vi "Acquire Waveform.vi"() -> ()   [LabVIEW 2020]
uses:
  Clients/NW and PSD_client/NW and PSD_client Class/NW and PSD_client.lvclass
panel:
  in  "Start Acquisition":bool
  in  "sine amplitude":dbl=1.0 format="%#.6g"
  in  "sine frequency":dbl=1.0 format="%#.6g"
  in  "sampling info":cluster{"Fs":dbl, "#s":dbl}={"Fs"=1000.0, "#s"=10000.0} {"#s" format="%#.6g"; "Fs" format="%#.6g"}
  out "Waveform":sgl[](graph)
  # "Waveform Parameters"
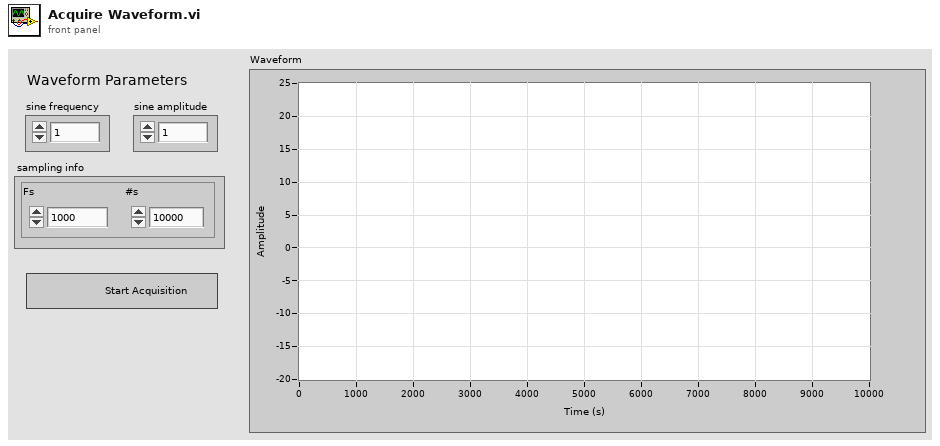
[diagram p1: front panel]
types:
  T1 = cluster{"sine frequency":dbl, "sine amplitude":dbl, "sampling info":cluster{"Fs":dbl, "#s":dbl}, "Start Acquisition?":bool}
  T2 = typedef "NW and PSD_client.lvlib/NW and PSD_client.lvclass/example_SignalData_Data.ctl" = cluster{"samples":sgl[]}
  T3 = cluster{"sampling info":cluster{"Fs":dbl, "#s":dbl}, "sine frequency":dbl, "sine amplitude":dbl}
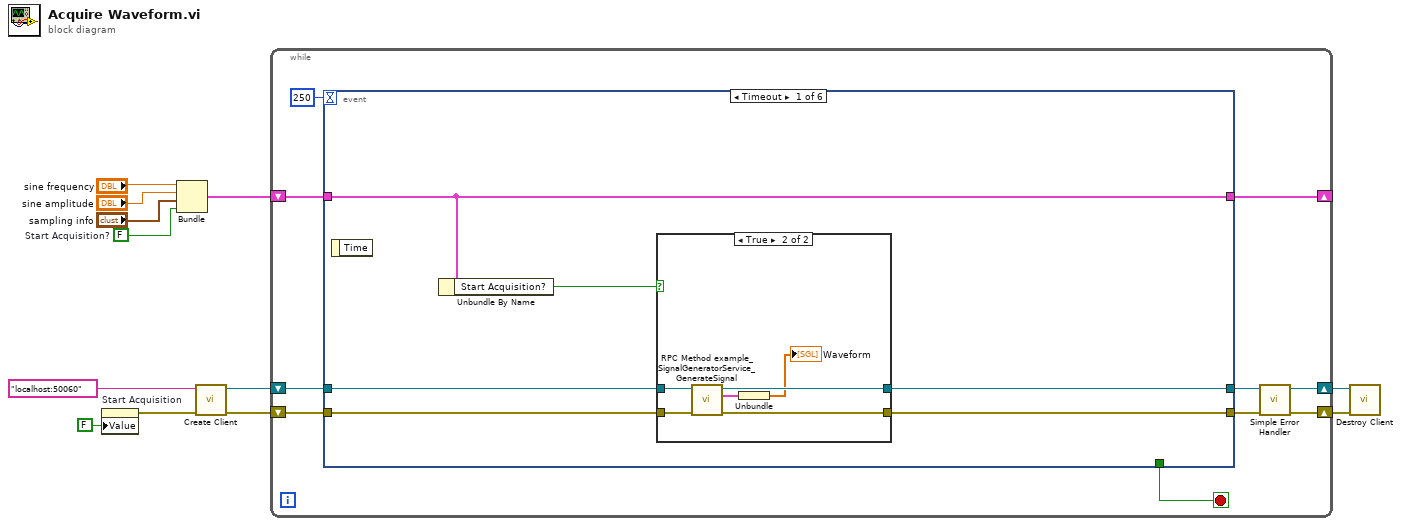
[diagram p0: block diagram]
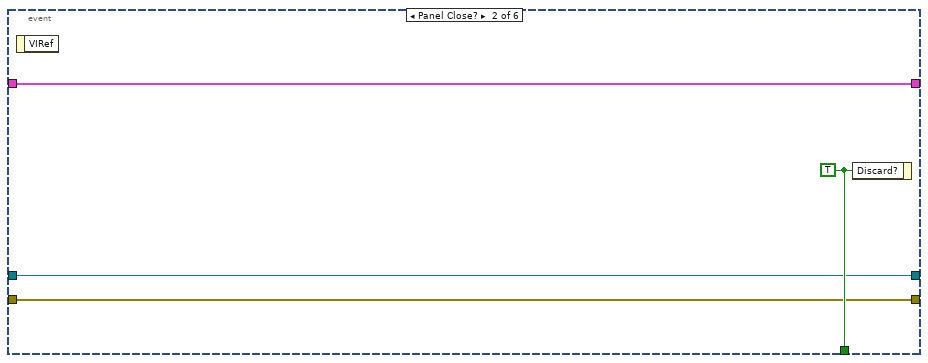
[diagram p3: hidden frame]
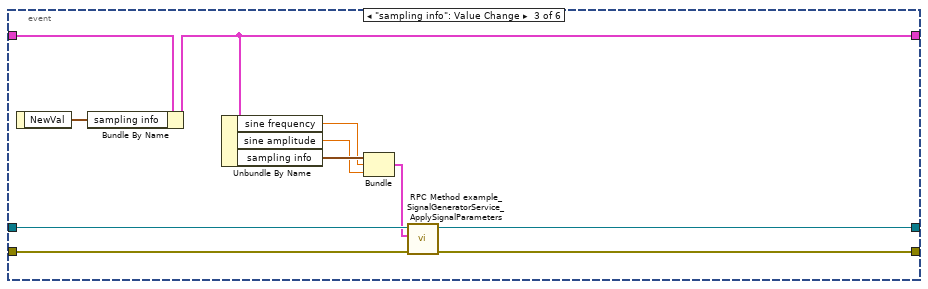
[diagram p4: hidden frame]
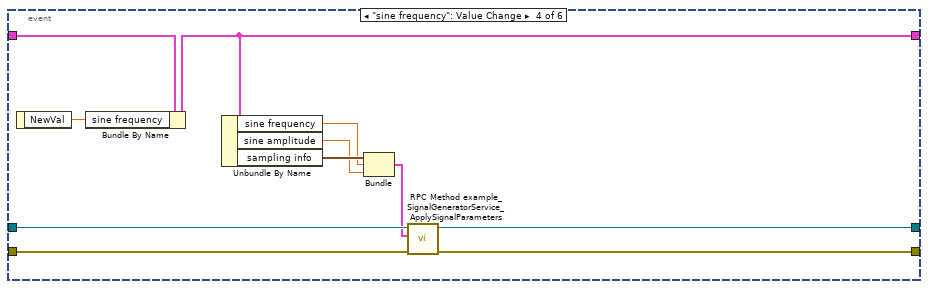
[diagram p5: hidden frame]
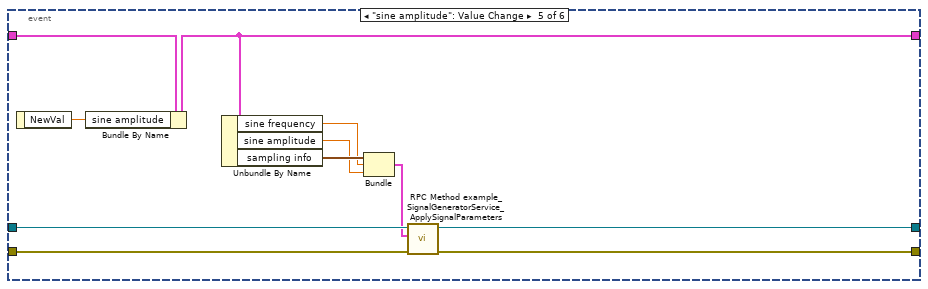
[diagram p6: hidden frame]
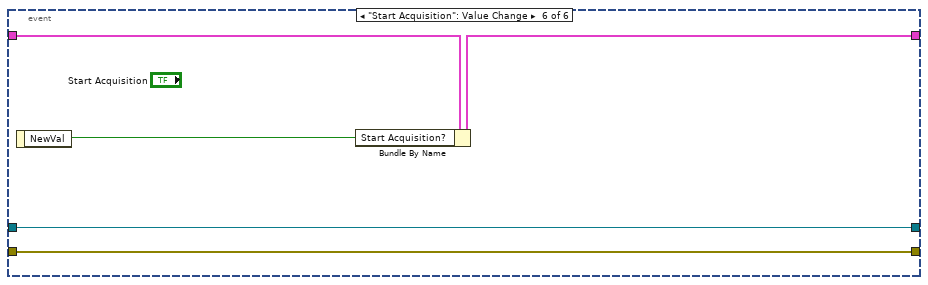
[diagram p7: hidden frame]
diagram:
  w4 = FALSE  # Start Acquisition?
  n1 = property on="Start Acquisition" class="Bool (strict)"("Value"=FALSE ("Start Acquisition")) -> (error out=w1:errorcluster)  [unwired: 2 in, 1 out]
  n2 = Bundle("sine frequency"="sine frequency", "sine amplitude"="sine amplitude", "sampling info"="sampling info", "Start Acquisition?"=w4) -> (w9:T1)  [unwired: 1 in]
  n3 = call "Create Client.vi"("error in (no error)"=w1, "address"="localhost:50060") -> ("error out"=w7:errorcluster, "gRPC Client out"=w8:refnum<class "NW and PSD_client.lvclass">)  [unwired: 8 in]
  n4 = while {
    shift-right: [w20] -> _
    shift-left: w9 -> [w21]
    shift-right: [w17] -> w6
    shift-left: w8 -> [w19]
    shift-right: [w15] -> w5
    shift-left: w7 -> [w18]
    stop <- w14 stop-if-true
    n5 = event shown="[0] Timeout" {
      selector: _ -> [_ _ _ _ _ _]
      dyn-events: _ -> [_ _ _ _ _ _]
      timeout: 250 -> [_ _ _ _ _ _]
      tunnel: w21 -> [w27 w39 w50 w61 w72 w73]
      tunnel: [w27 w39 w44 w55 w66 w74] -> w20
      tunnel: w19 -> [w26 w36 w48 w59 w70 w77]
      tunnel: w18 -> [w23 w37 w46 w57 w68 w76]
      tunnel: [w25 w36 w47 w58 w69 w77] -> w17
      tunnel: [w24 w37 w45 w56 w67 w76] -> w16
      tunnel: [_ w38 _ _ _ _] -> w14
      event Timeout {
        n6 = event-data() -> ()  [unwired: 1 in, 1 out]
        n7 = Unbundle By Name(w27) -> ("Start Acquisition?"=w22:bool)
        n8 = case shown="True" w22 {
          tunnel: w26 -> [w29 w35]
          tunnel: [w29 w34] -> w25
          tunnel: [w28 w33] -> w24
          tunnel: w23 -> [w28 w32]
          frame False {
          }
          frame True {
            n9 = call "RPC Method example_SignalGeneratorService_GenerateSignal.vi"("error in (no error)"=w32, "gRPC Client in"=w35) -> ("error out"=w33:errorcluster, "Response Data"=w31:T2, "gRPC Client out"=w34:refnum<class "NW and PSD_client.lvclass">)  [unwired: 7 in]
            n10 = Unbundle(w31) -> ("samples"=→"Waveform":sgl[])
          }
        }
      }
      event Panel Close? {
        w38 = TRUE ("Discard?")
        n11 = event-data() -> ()  [unwired: 1 in, 1 out]
        n12 = event-data("Discard?"=w38) -> ()  [unwired: 1 in, 1 out]
      }
      event "sampling info": Value Change {
        n13 = event-data() -> ("NewVal"=w49:cluster{"Fs":dbl, "#s":dbl})  [unwired: 1 in]
        n14 = Bundle By Name(cluster=w50, "sampling info"=w49) -> (w44:T1)
        n15 = Unbundle By Name(w44) -> ("sine frequency"=w42:dbl, "sine amplitude"=w41:dbl, "sampling info"=w43:cluster{"Fs":dbl, "#s":dbl})
        n16 = Bundle("sampling info"=w43, "sine frequency"=w42, "sine amplitude"=w41) -> (w40:T3)  [unwired: 1 in]
        n17 = call "RPC Method example_SignalGeneratorService_ApplySignalParameters.vi"("error in (no error)"=w46, "Request Data"=w40, "gRPC Client in"=w48) -> ("error out"=w45:errorcluster, "gRPC Client out"=w47:refnum<class "NW and PSD_client.lvclass">)  [unwired: 6 in, 1 out]
      }
      event "sine frequency": Value Change {
        n18 = event-data() -> ("NewVal"=w60:dbl)  [unwired: 1 in]
        n19 = Bundle By Name(cluster=w61, "sine frequency"=w60) -> (w55:T1)
        n20 = Unbundle By Name(w55) -> ("sine frequency"=w53:dbl, "sine amplitude"=w52:dbl, "sampling info"=w54:cluster{"Fs":dbl, "#s":dbl})
        n21 = Bundle("sampling info"=w54, "sine frequency"=w53, "sine amplitude"=w52) -> (w51:T3)  [unwired: 1 in]
        n22 = call "RPC Method example_SignalGeneratorService_ApplySignalParameters.vi"("error in (no error)"=w57, "Request Data"=w51, "gRPC Client in"=w59) -> ("error out"=w56:errorcluster, "gRPC Client out"=w58:refnum<class "NW and PSD_client.lvclass">)  [unwired: 6 in, 1 out]
      }
      event "sine amplitude": Value Change {
        n23 = event-data() -> ("NewVal"=w71:dbl)  [unwired: 1 in]
        n24 = Bundle By Name(cluster=w72, "sine amplitude"=w71) -> (w66:T1)
        n25 = Unbundle By Name(w66) -> ("sine frequency"=w64:dbl, "sine amplitude"=w63:dbl, "sampling info"=w65:cluster{"Fs":dbl, "#s":dbl})
        n26 = Bundle("sampling info"=w65, "sine frequency"=w64, "sine amplitude"=w63) -> (w62:T3)  [unwired: 1 in]
        n27 = call "RPC Method example_SignalGeneratorService_ApplySignalParameters.vi"("error in (no error)"=w68, "Request Data"=w62, "gRPC Client in"=w70) -> ("error out"=w67:errorcluster, "gRPC Client out"=w69:refnum<class "NW and PSD_client.lvclass">)  [unwired: 6 in, 1 out]
      }
      event "Start Acquisition": Value Change {
        n28 = event-data() -> ("NewVal"=w75:bool)  [unwired: 1 in]
        n29 = Bundle By Name(cluster=w73, "Start Acquisition?"=w75) -> (w74:T1)
      }
    }
    n30 = call <vilib>:"Simple Error Handler.vi"("error in (no error)"=w16) -> ("error out"=w15:errorcluster)  [unwired: 4 in, 4 out]
  }
  n31 = call "Destroy Client.vi"("error in (no error)"=w5, "gRPC Client in"=w6) -> ()  [unwired: 8 in, 2 out]
